vi "Looping Chart Array Helper.vi"(9 "Datapoint In":dbl, 11 "Array from Loop":dbl[](array[numeric])) -> (0 "Processed Datapoint":dbl, 3 "Array to Loop":dbl[](array[numeric]), 4 "Data Array to Chart":dbl[](array[numeric]))   [LabVIEW 2021]
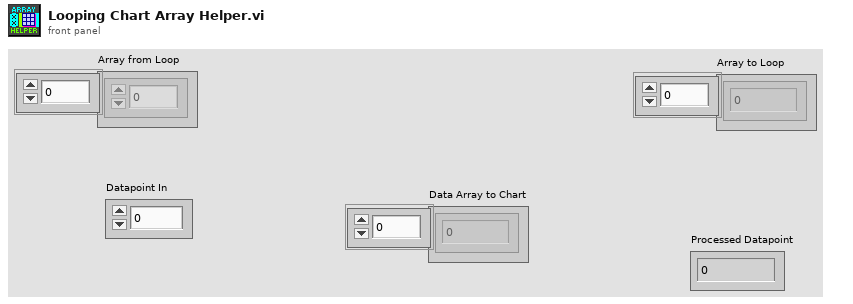
[diagram p1: front panel]
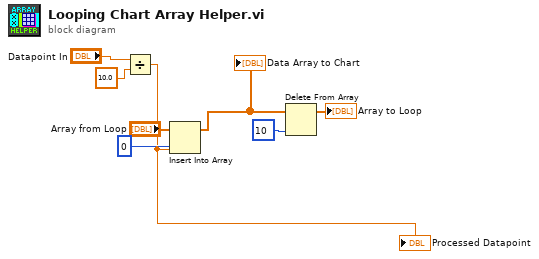
[diagram p0: block diagram]
diagram:
  n1 = Divide(x="Datapoint In", y=10.0) -> (x/y=w1:dbl)
  "Processed Datapoint" <- w1
  n2 = Insert Into Array(array="Array from Loop", index=0, new element=w1) -> (w5:dbl[])
  "Data Array to Chart" <- w5
  n3 = Delete From Array(array=w5, index=10) -> (array with subset deleted=→"Array to Loop":dbl[])  [unwired: 1 in, 1 out]
